vi "TeleopAutoBalance.vi"(10 "Match Info":T1={"Autonomous Elapsed Seconds"=0.0, "TeleOp Elapsed Seconds"=0.0, "Disabled Elapsed Seconds"=0.0, "Visited Autonomous"=FALSE, "Visited TeleOp"=FALSE, "Visited Disabled"=FALSE, "Autonomous Settings"={"Autonomous Style"=enum."Independent", "VI Refnum"=refnum}}, 11 "Call Context":T2) -> ()   [LabVIEW 2016]
doc: "This VI is called for each TeleOp packet received from the DS where the robot is not disabled. It is often used to read from the joysticks and update I/O or to update setpoints for timed control loops. It should complete and return within 20 milliseconds or it may miss DS packets."
uses:
  <vilib>/Rock Robotics/WPI/DriverStation/WPI_DriverStationDerivedRobotMode.ctl
  <vilib>/Rock Robotics/WPI/DriverStation/WPI_DriverStationMatch Info.ctl
  <vilib>/Rock Robotics/WPI/Utilities/WPI_GetSetVariantRefNum.vi
  <vilib>/Rock Robotics/Network Tables/SD Write Boolean Array.vi
  <vilib>/Rock Robotics/Network Tables/SD Write Numeric Array.vi
  <vilib>/Rock Robotics/Network Tables/SD Read Boolean.vi
  <vilib>/Rock Robotics/Network Tables/SD Read Number.vi
  <vilib>/Rock Robotics/WPI/RobotDrive/WPI_RobotDriveMecanumDrive_Cartesian.vi
panel:
  out "Sample Slider 0":dbl(slide) scale=0.0..5.0
  out "Sample Boolean 1":bool
  out "Sample Boolean 0":bool
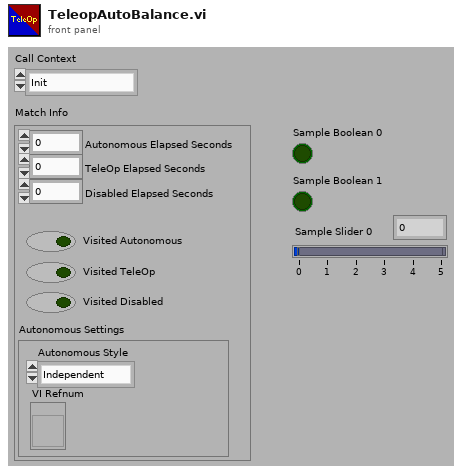
[diagram p1: front panel]
types:
  T1 = typedef "WPI_DriverStationMatch Info.ctl" = cluster{"Autonomous Elapsed Seconds":dbl, "TeleOp Elapsed Seconds":dbl, "Disabled Elapsed Seconds":dbl, "Visited Autonomous":bool, "Visited TeleOp":bool, "Visited Disabled":bool, "Autonomous Settings":cluster{"Autonomous Style":enum16{"Iterative", "Independent"}, "VI Refnum":refnum<vi>}}
  T2 = typedef "WPI_DriverStationDerivedRobotMode.ctl" = enum16{"Init", "Execute", "Stop"}
  T3 = typedef "WPI_JoystickDevRef.ctl" = cluster{"Device":T4}
  T4 = typedef "WPI_JoystickDeviceEnum.ctl" = enum16{"USB 0", "USB 1", "USB 2", "USB 3", "USB 4", "USB 5"}
  T5 = typedef "WPI_RobotDriveDevRef.ctl" = cluster{"DevStatus":errorcluster, "Motors[]":T6[], "Square Inputs":bool, "Max Output":dbl}
  T6 = typedef "WPI_MotorControlDeviceRef.ctl" = cluster{"DeviceStatus":errorcluster, "Type":T7, "PWM":cluster{"PWM Channel":T8, "DeadBand":T9}, "CAN":cluster{"Device Number":u8, "SetOutput VI Ref":variant, "GetOutput VI Ref":variant, "Enable VI Ref":variant, "Disable VI Ref":variant, "Data":variant}, "Invert":bool}
  T7 = typedef "WPI_MotorControlType.ctl" = enum16{"PWM", "CAN"}
  T8 = typedef "FPGA_DIOPWMChannel.ctl" = enum8{"PWM 0", "PWM 1", "PWM 2", "PWM 3", "PWM 4", "PWM 5", "PWM 6", "PWM 7", "PWM 8", "PWM 9", "PWM MXP 0", "PWM MXP 1", "PWM MXP 2", "PWM MXP 3", "PWM MXP 4", "PWM MXP 5", "PWM MXP 6", "PWM MXP 7", "PWM MXP 8", "PWM MXP 9", "Invalid"}
  T9 = typedef "WPI_PWMDeadband.ctl" = cluster{"Name":string, "maxPositivePwm":i32, "minPositivePwm":i32, "centerPwm":i32, "maxNegativePwm":i32, "minNegativePwm":i32, "angularRange":u16}
  T10 = cluster{"Yaw":dbl, "Roll":dbl, "Pitch":dbl, "Heading":dbl, "Fused Heading":dbl}
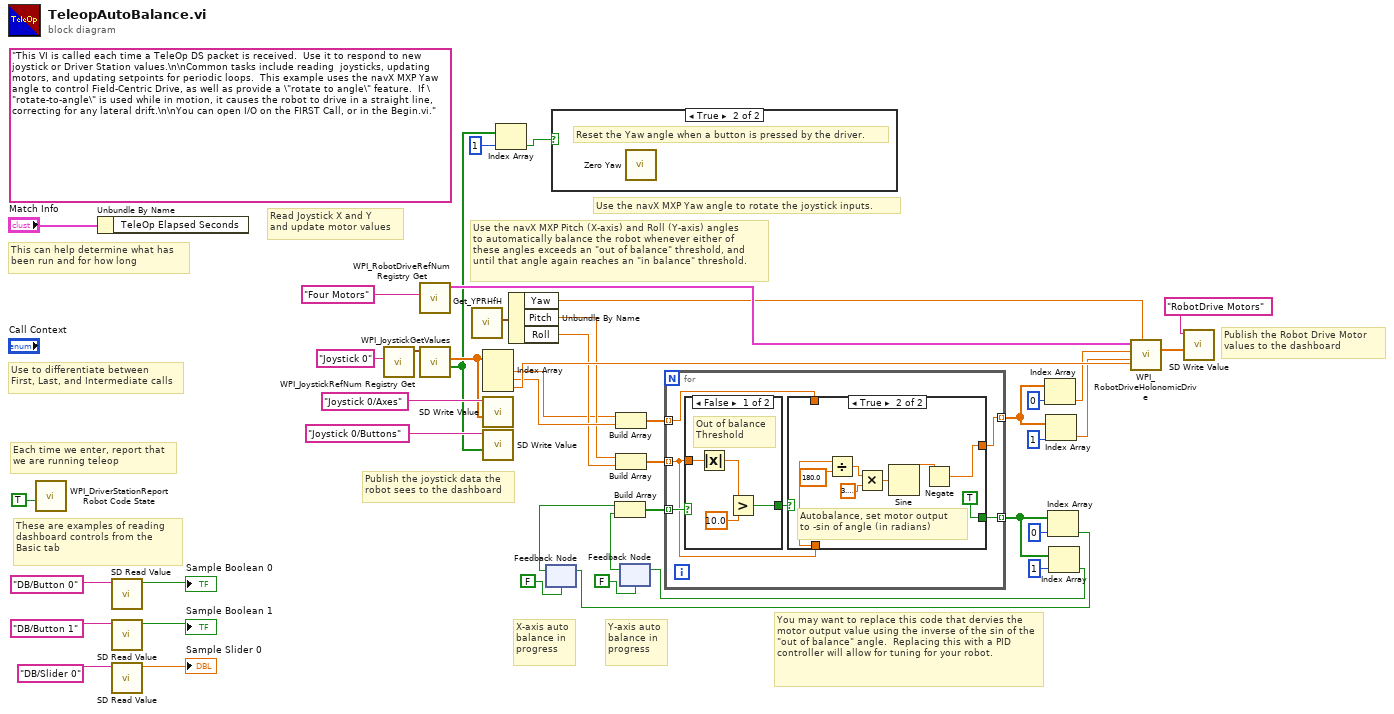
[diagram p0: block diagram]
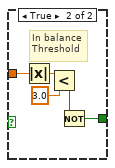
[diagram p3: hidden frame]
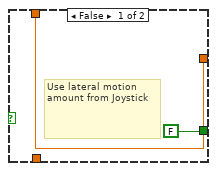
[diagram p4: hidden frame]
diagram:
  (unwired) "This VI is called each time a TeleOp DS packet is received.  Use it to respond to new joystick or Driver Station values.\n\nCommon tasks include reading  joysticks, updating motors, and updating setpoints for periodic loops.  This example uses the navX MXP Yaw angle to control Field-Centric Drive, as well as provide a \"rotate to angle\" feature.  If \"rotate-to-angle\" is used while in motion, it causes the robot to drive in a straight line, correcting for any lateral drift.\n\nYou can open I/O on the FIRST Call, or in the Begin.vi."
  # "You may want to replace this code that dervies the motor output value using the inverse of the sin of the \"out of balance\" angle.  Replacing this with a PID controller will allow for tuning for your robot."
  # "Y-axis auto\nbalance in \nprogress"
  # "X-axis auto\nbalance in \nprogress"
  # "Use the navX MXP Pitch (X-axis) and Roll (Y-axis) angles\nto automatically balance the robot whenever either of \nthese angles exceeds an \"out of balance\" threshold, and\nuntil that angle again reaches an \"in balance\" threshold."
  # "Use the navX MXP Yaw angle to rotate the joystick inputs."
  # "These are examples of reading dashboard controls from the Basic tab"
  # "Publish the Robot Drive Motor\nvalues to the dashboard"
  # "Publish the joystick data the\nrobot sees to the dashboard"
  # "Each time we enter, report that\nwe are running teleop"
  # "Use to differentiate between\nFirst, Last, and Intermediate calls"
  # "This can help determine what has\nbeen run and for how long"
  # "Read Joystick X and Y \nand update motor values"
  n1 = call <vilib>:"WPI_DriverStationReport Robot Code State.vi"("TeleOp"=TRUE ("Autonomous")) -> ()  [unwired: 10 in, 1 out]
  n2 = Unbundle By Name("Match Info") -> ()  [unwired: 1 out]
  n3 = call-poly <vilib>:"SD Read Value.vi"("Name"="DB/Button 0" ("refnum name")) -> ("Boolean"=→"Sample Boolean 0":bool)  [unwired: 8 in, 2 out]
  n4 = call-poly <vilib>:"SD Read Value.vi"("Name"="DB/Button 1" ("refnum name")) -> ("Boolean"=→"Sample Boolean 1":bool)  [unwired: 8 in, 2 out]
  n5 = call-poly <vilib>:"SD Read Value.vi"("Name"="DB/Slider 0" ("refnum name")) -> ("Numeric"=→"Sample Slider 0":dbl)  [unwired: 8 in, 2 out]
  n6 = call <vilib>:"WPI_JoystickRefNum Registry Get.vi"("refnum name"="Joystick 0") -> ("JoystickDevRef"=w40:T3)  [unwired: 1 in, 9 out]
  n7 = call <vilib>:"WPI_RobotDriveRefNum Registry Get.vi"("refnum name"="Four Motors") -> ("RobotDriveDevRef"=w42:T5)  [unwired: 1 in, 9 out]
  n8 = call <vilib>:"WPI_JoystickGetValues.vi"("JoystickDevRef"=w40) -> ("Buttons"=w25:bool[], "Axes"=w28:dbl[])  [unwired: 6 in, 3 out]
  n9 = call "Get_YPRHfH.vi"() -> ("YRPHfH"=w1:T10)  [unwired: 11 in]
  n10 = Index Array(array=w28) -> (element #1=w3:dbl, element #2=w7:dbl, element #3=w24:dbl)  [unwired: 3 in]
  n11 = call-poly <vilib>:"SD Write Value.vi"("Numeric Array"=w28, "Name"="Joystick 0/Axes") -> ()  [unwired: 8 in, 2 out]
  n12 = call-poly <vilib>:"SD Write Value.vi"("Boolean Array"=w25, "Name"="Joystick 0/Buttons") -> ()  [unwired: 8 in, 2 out]
  n13 = Index Array(array=w25, index=1) -> (element=w2:bool)
  n14 = Unbundle By Name(w1) -> ("Yaw"=w26:dbl, "Pitch"=w6:dbl, "Roll"=w5:dbl)
  n15 = feedback #1(FALSE) -> (w21:bool)
  n16 = case shown="True" w2 {
    frame False {
    }
    frame True {
      # "Reset the Yaw angle when a button is pressed by the driver."
      n17 = call "Zero Yaw.vi"() -> ()  [unwired: 12 in]
    }
  }
  n18 = Build Array(w3, w7) -> (w18:dbl[])
  n19 = Build Array(w6, w5) -> (w4:dbl[])
  n20 = feedback #2(FALSE) -> (w20:bool)
  n21 = Build Array(w21, w20) -> (w19:bool[])
  n22 = for {
    tunnel: w19 -> [w49] mode=indexing
    tunnel: w18 -> [w45] mode=indexing
    tunnel: [w48] -> w17 mode=indexing
    tunnel: [w47] -> w10 mode=indexing
    tunnel: w4 -> [w46] mode=indexing
    n23 = case shown="False" w49 {
      tunnel: w46 -> [w54 w57]
      tunnel: [w51 w56] -> w50
      frame False {
        # "Out of balance\nThreshold"
        n24 = Absolute Value(x=w54) -> (abs(x)=w53:dbl)
        n25 = Greater?(x=w53, y=10.0) -> (0:w51:bool)
      }
      frame True {
        # "In balance\nThreshold"
        n26 = Absolute Value(x=w57) -> (abs(x)=w58:dbl)
        n27 = Less?(x=w58, y=3.0) -> (x < y?=w55:bool)
        n28 = Not(x=w55) -> (.not. x?=w56:bool)
      }
    }
    n29 = case shown="True" w50 {
      tunnel: w46 -> [_ w68]
      tunnel: [w60 w62] -> w47
      tunnel: [FALSE TRUE] -> w48
      tunnel: w45 -> [w60 _]
      frame False {
        # "Use lateral motion amount from Joystick"
      }
      frame True {
        # "Autobalance, set motor output \nto -sin of angle (in radians)"
        n30 = Divide(x=w68, y=180.0) -> (x/y=w66:dbl)
        n31 = Multiply(x=w66, y=3.141592653589793) -> (x*y=w64:dbl)
        n32 = Sine(x=w64) -> (sin(x)=w63:dbl)
        n33 = Negate(x=w63) -> (-x=w62:dbl)
      }
    }
  }
  n34 = Index Array(array=w10, index=0) -> (element=w9:dbl)
  n35 = Index Array(array=w10, index=1) -> (element=w8:dbl)
  n36 = Index Array(array=w17, index=0) -> (element=w14:bool)
  n37 = feedback-in #1(w14) -> ()
  n38 = Index Array(array=w17, index=1) -> (element=w13:bool)
  n39 = feedback-in #2(w13) -> ()
  n40 = call-poly <vilib>:"WPI_RobotDriveHolonomicDrive.vi"("Rotation"=w24, "Gyro Angle"=w26, "Y"=w8, "X"=w9, "RobotDriveDevRef"=w42) -> ("Motor Values"=w29:dbl[])  [unwired: 4 in, 2 out]
  n41 = call-poly <vilib>:"SD Write Value.vi"("Numeric Array"=w29, "Name"="RobotDrive Motors") -> ()  [unwired: 8 in, 2 out]
